vi "TX OOB Test Cases.vi"() -> (0 "error out":errorcluster, 2 "status":string, 3 "pass":bool)   [LabVIEW 2021]
uses:
  CIFCoreCommon/Typedef/Plugin Status.ctl
  CIFCoreCommon/Typedef/Plugin State.ctl
  CIFCoreCommon/Typedef/Timing Statistics.ctl
  CIFCoreCommon/Typedef/Timing Stats Base.ctl
  CIFCoreCommon/Typedef/FIFO Statistics.ctl
  CIFCoreCommon/Typedef/Simple Error.ctl
  CIFCoreCommon/Typedef/Monitor Doubles.ctl
  CIFCoreCommon/Typedef/Monitor U64.ctl
  CIFCoreCommon/Typedef/Monitor I64.ctl
  CIFUtilities/CIFOutOfBand/CIFOutOfBand.lvclass/CIFOutOfBand.ctl
  OOB_Tx/Typedef/OOB Core Commands.ctl
  CIFCoreCommon/Typedef/Plugin Overrides.ctl
  CIFCoreCommon/Typedef/Timing Overrides.ctl
  OOB_Tx/Private/Command Settings.vi
  CIFUtilities/CIFOutOfBand/Accessors/Write Local OOB Data.vi
  CIFUtilities/CIFOutOfBand/Write OOB DVR.vi
  CIFUtilities/CIFOutOfBand/Utilities/Command to Bitwise Command.vi
  CIFUtilities/CIFOutOfBand/Accessors/Read Local OOB Data.vi
  CIFUtilities/CIFOutOfBand/Read OOB DVR.vi
  OOB_Tx/Private/Read Payload.vi
  OOB_Tx/CIFCoreOOB_Tx.lvclass
  D:/dev/CIF-LVCore/src/CIFUtilities/CIFOutOfBand/CIFOutOfBand.lvclass
  CIFUtilities/CIFOutOfBand/Init OOB.vi
  CIFUtilities/CIFOutOfBand/CIFOutOfBand.lvclass
  CIFCoreCommon/CIFCoreCommon.lvlib
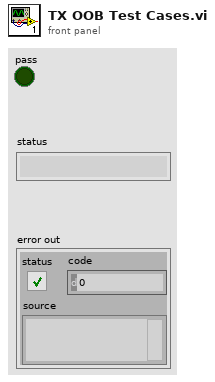
[diagram p1: front panel]
types:
  T1 = typedef "CIFCoreCommon.lvlib/Plugin Status.ctl" = cluster{"State":T2, "Timing Statistics (us)":T3, "FIFO Statistics (us)":T5, "error":T6, "Monitor Doubles":T7, "Monitor U64":T8, "Monitor I64":T9}
  T2 = typedef "CIFCoreCommon.lvlib/Plugin State.ctl" = enum32{"Null", "Creating", "Listening", "Running", "CleaningUp", "Destroying"}
  T3 = typedef "CIFCoreCommon.lvlib/Timing Statistics.ctl" = cluster{"Period":T4, "Wake Error":T4, "Execute":T4, "Housekeep":T4, "Idle":T4}
  T4 = typedef "CIFCoreCommon.lvlib/Timing Stats Base.ctl" = cluster{"Max":i32, "Min":i32}
  T5 = typedef "CIFCoreCommon.lvlib/FIFO Statistics.ctl" = cluster{"From T0":T4, "From Previous Plugin":T4, "Output Error":T4}
  T6 = typedef "CIFCoreCommon.lvlib/Simple Error.ctl" = cluster{"status":bool, "code":i32}
  T7 = typedef "CIFCoreCommon.lvlib/Monitor Doubles.ctl" = cluster{"1":dbl, "2":dbl, "3":dbl, "4":dbl}
  T8 = typedef "CIFCoreCommon.lvlib/Monitor U64.ctl" = cluster{"1":u64, "2":u64, "3":u64, "4":u64}
  T9 = typedef "CIFCoreCommon.lvlib/Monitor I64.ctl" = cluster{"1":i64, "2":i64, "3":i64, "4":i64}
  T10 = typedef "CIFCoreOOB_Tx.lvclass/OOB Core Commands.ctl" = enum8{"Status", "Overrides"}
  T11 = typedef "CIFCoreCommon.lvlib/Plugin Overrides.ctl" = cluster{"Timing Overrides":T12}
  T12 = typedef "CIFCoreCommon.lvlib/Timing Overrides.ctl" = cluster{"Override Timing":bool, "Period (s)":dbl}
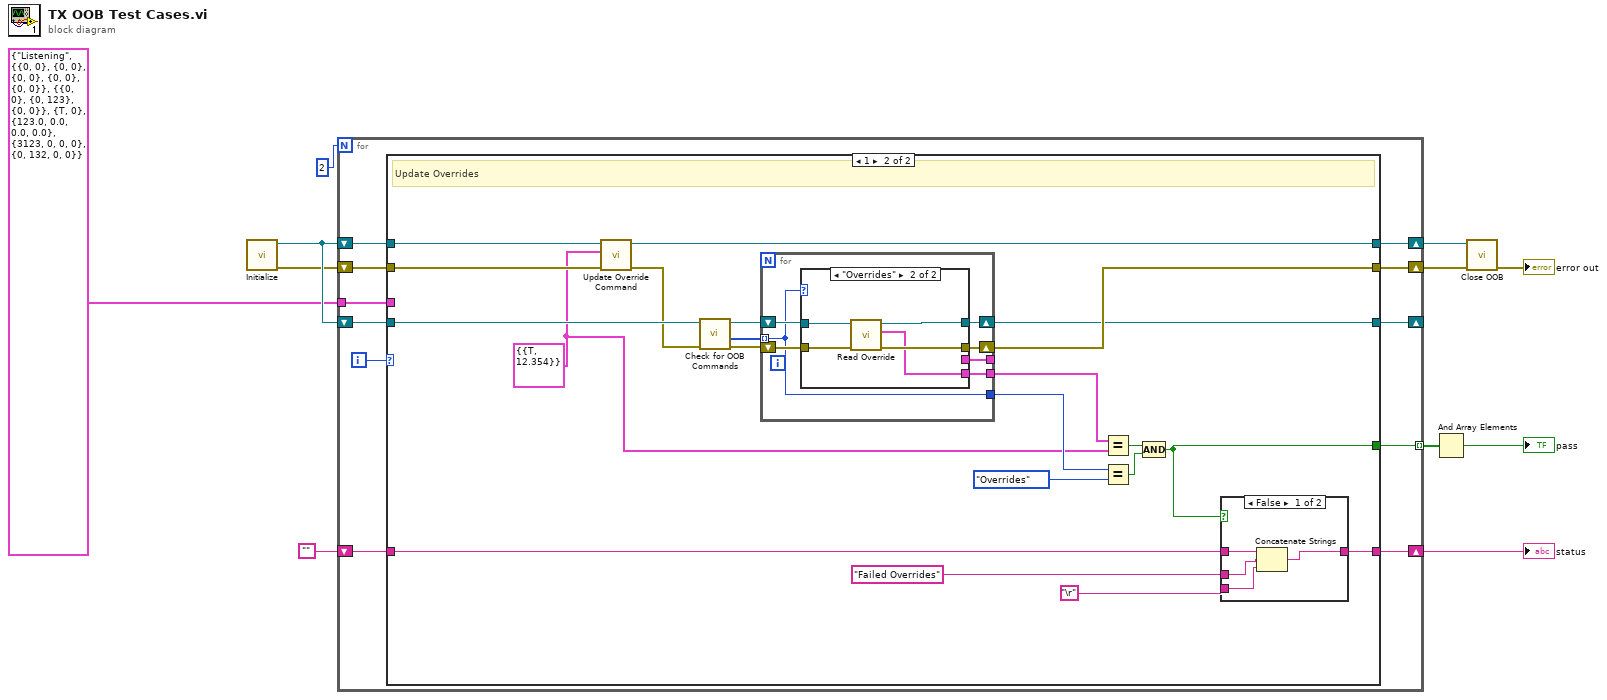
[diagram p0: block diagram]
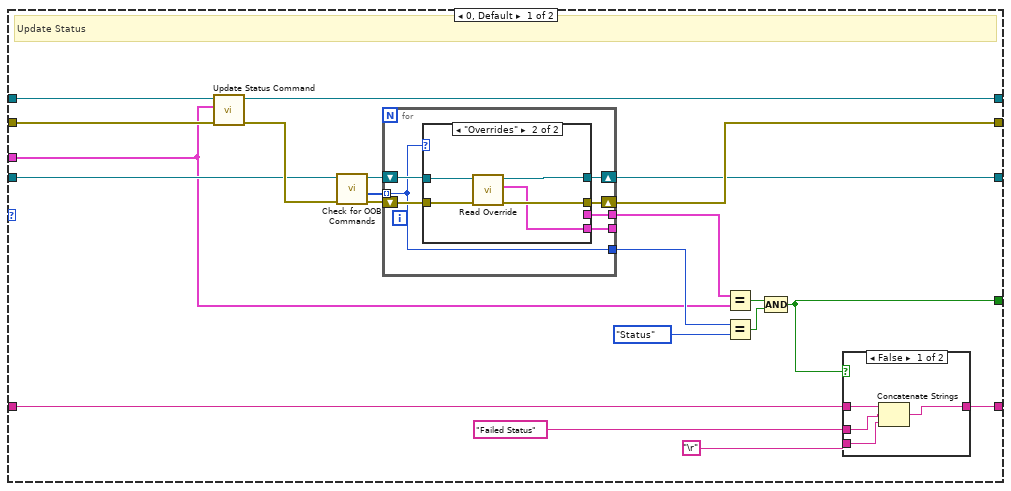
[diagram p2: hidden frame]
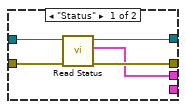
[diagram p3: hidden frame]
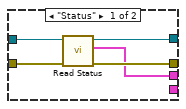
[diagram p5: hidden frame]
diagram:
  n1 = call "Initialize.vi"() -> ("error out"=w2:errorcluster, "CoreOOB_Tx out"=w3:refnum<class "CIFCoreOOB_Tx.lvclass">)  [unwired: 10 in]
  n2 = for {
    N: 2 -> [_]
    tunnel: [w22] -> w9 mode=indexing
    shift-right: [w19] -> w10
    shift-left: w2 -> [w21]
    shift-right: [w13] -> w11
    shift-left: w3 -> [w20]
    shift-right: [w12] -> _
    shift-left: w3 -> [w17]
    shift-right: [w15] -> w6
    shift-left: "" -> [w16]
    tunnel: T1 {"State"=enum."Listening", "Timing Statistics (us)"={"Period"={"Max"=0, "Min"=0}, "Wake Error"={"Max"=0, "Min"=0}, "Execute"={"Max"=0, "Min"=0}, "Housekeep"={"Max"=0, "Min"=0}, "Idle"={"Max"=0, "Min"=0}}, "FIFO Statistics (us)"={"From T0"={"Max"=0, "Min"=0}, "From Previous Plugin"={"Max"=0, "Min"=123}, "Output Error"={"Max"=0, "Min"=0}}, "error"={"status"=TRUE, "code"=0}, "Monitor Doubles"={"1"=123.0, "2"=0.0, "3"=0.0, "4"=0.0}, "Monitor U64"={"1"=3123, "2"=0, "3"=0, "4"=0}, "Monitor I64"={"1"=0, "2"=132, "3"=0, "4"=0}} ("Status") -> [w14]
    i -> [w18]
    n3 = case shown="1" w18 {
      tunnel: [w35 w78] -> w22
      tunnel: w21 -> [w30 w69]
      tunnel: w20 -> [w32 w70]
      tunnel: [w43 w86] -> w19
      tunnel: [w31 w67] -> w13
      tunnel: w17 -> [w28 w76]
      tunnel: [w42 w85] -> w12
      tunnel: w16 -> [w41 w84]
      tunnel: [w40 w83] -> w15
      tunnel: w14 -> [w24 _]
      frame 0, Default {
        # "Update Status"
        n4 = call "Update Status Command.vi"("error in"=w30, "Status"=w24, "CoreOOB_Tx in"=w32) -> ("error out"=w29:errorcluster, "CoreOOB_Tx out"=w31:refnum<class "CIFCoreOOB_Tx.lvclass">)  [unwired: 7 in]
        n5 = call "Check for OOB Commands.vi"("error in (no error)"=w29, "CoreOOB_Tx in"=w28) -> ("error out"=w27:errorcluster, "Commands"=w25:T10[], "CoreOOB_Tx out"=w26:refnum<class "CIFCoreOOB_Tx.lvclass">)  [unwired: 6 in, 1 out]
        n6 = for {
          tunnel: w25 -> [w45] mode=indexing
          shift-right: [w50] -> w43
          shift-left: w27 -> [w48]
          shift-right: [w49] -> w42
          shift-left: w26 -> [w47]
          tunnel: [w46] -> w34
          tunnel: [w45] -> w33
          tunnel: [w44] -> _
          n7 = case shown="\"Overrides\"" w45 {
            tunnel: w47 -> [w55 w59]
            tunnel: w48 -> [w54 w60]
            tunnel: [w53 w58] -> w49
            tunnel: [w52 w57] -> w50
            tunnel: [w51 _] -> w46
            tunnel: [_ w56] -> w44
            frame "Status" {
              n8 = call "Read Status.vi"("error in"=w54, "CoreOOB_Tx in"=w55) -> ("error out"=w52:errorcluster, "Status"=w51:T1, "CoreOOB_Tx out"=w53:refnum<class "CIFCoreOOB_Tx.lvclass">)  [unwired: 7 in]
            }
            frame "Overrides" {
              n9 = call "Read Override.vi"("error in"=w60, "CoreOOB_Tx in"=w59) -> ("error out"=w57:errorcluster, "Plugin Overrides"=w56:T11, "CoreOOB_Tx out"=w58:refnum<class "CIFCoreOOB_Tx.lvclass">)  [unwired: 7 in]
            }
          }
        }
        n10 = Equal?(x=w34, y=w24) -> (x = y?=w37:bool)
        n11 = Equal?(x=w33, y=OOB_Core_Commands."Status") -> (x = y?=w36:bool)
        n12 = Compound Arithmetic op=AND(w37, w36) -> (w35:bool)
        n13 = case shown="False" w35 {
          tunnel: w41 -> [w64 w65]
          tunnel: [w61 w65] -> w40
          tunnel: "Failed Status" -> [w63 _]
          tunnel: "\r" -> [w62 _]
          frame False {
            n14 = Concatenate Strings(w64, w63, w62) -> (w61:string)
          }
          frame True {
          }
        }
      }
      frame 1 {
        w66 = T11 {"Timing Overrides"={"Override Timing"=TRUE, "Period (s)"=12.354}} ("Plugin Overrides")
        # "Update Overrides"
        n15 = call "Update Override Command.vi"("error in"=w69, "Plugin Overrides"=w66, "CoreOOB_Tx in"=w70) -> ("error out"=w68:errorcluster, "CoreOOB_Tx out"=w67:refnum<class "CIFCoreOOB_Tx.lvclass">)  [unwired: 7 in]
        n16 = call "Check for OOB Commands.vi"("error in (no error)"=w68, "CoreOOB_Tx in"=w76) -> ("error out"=w75:errorcluster, "Commands"=w73:T10[], "CoreOOB_Tx out"=w74:refnum<class "CIFCoreOOB_Tx.lvclass">)  [unwired: 6 in, 1 out]
        n17 = for {
          tunnel: w73 -> [w88] mode=indexing
          shift-right: [w93] -> w86
          shift-left: w75 -> [w91]
          shift-right: [w92] -> w85
          shift-left: w74 -> [w90]
          tunnel: [w89] -> _
          tunnel: [w88] -> w77
          tunnel: [w87] -> w71
          n18 = case shown="\"Overrides\"" w88 {
            tunnel: w90 -> [w98 w102]
            tunnel: w91 -> [w97 w103]
            tunnel: [w96 w101] -> w92
            tunnel: [w95 w100] -> w93
            tunnel: [w94 _] -> w89
            tunnel: [_ w99] -> w87
            frame "Status" {
              n19 = call "Read Status.vi"("error in"=w97, "CoreOOB_Tx in"=w98) -> ("error out"=w95:errorcluster, "Status"=w94:T1, "CoreOOB_Tx out"=w96:refnum<class "CIFCoreOOB_Tx.lvclass">)  [unwired: 7 in]
            }
            frame "Overrides" {
              n20 = call "Read Override.vi"("error in"=w103, "CoreOOB_Tx in"=w102) -> ("error out"=w100:errorcluster, "Plugin Overrides"=w99:T11, "CoreOOB_Tx out"=w101:refnum<class "CIFCoreOOB_Tx.lvclass">)  [unwired: 7 in]
            }
          }
        }
        n21 = Equal?(x=w71, y=w66) -> (x = y?=w80:bool)
        n22 = Equal?(x=w77, y=OOB_Core_Commands."Overrides") -> (x = y?=w79:bool)
        n23 = Compound Arithmetic op=AND(w80, w79) -> (w78:bool)
        n24 = case shown="False" w78 {
          tunnel: w84 -> [w107 w108]
          tunnel: [w104 w108] -> w83
          tunnel: "Failed Overrides" -> [w106 _]
          tunnel: "\r" -> [w105 _]
          frame False {
            n25 = Concatenate Strings(w107, w106, w105) -> (w104:string)
          }
          frame True {
          }
        }
      }
    }
  }
  "status" <- w6
  n26 = And Array Elements(Boolean array=w9) -> (logical AND=→"pass":bool)
  n27 = call "Close OOB.vi"("error in"=w10, "OOB in"=w11) -> ("error out"=→"error out":errorcluster)  [unwired: 9 in]
